vi "Read XML_Parse BC messageBuffers.vi"(8 "error in (no error)":errorcluster, 10 "channel in":T1, 11 "busController in":refnum<k24>) -> (0 "error out":errorcluster, 2 "channel out":T1, 3 "busController out":refnum<k24>)   [LabVIEW 2020, in "Ballard 1553 System Explorer.lvlib"]
uses:
  Ballard 1553 System Explorer.lvlib
  Ballard_Channel.ctl
  Ballard_BC.ctl
  Ballard_message.ctl
  Ballard_messageType.ctl
  Ballard_CWD1.ctl
  Ballard_CWD2.ctl
  Ballard_minorFrame.ctl
  Ballard_majorFrame.ctl
  Ballard_acyclicFrame.ctl
  Ballard_RT.ctl
  Ballard_RT subAddress.ctl
  Ballard_RT direction.ctl
  Ballard_RT rtMode.ctl
  Ballard_RT modeCode.ctl
  C:/Users/Administrator/Desktop/GIT/Ballard-MIL-STD-1553-Custom-Device/Source/System Explorer/SubVIs/Parse XML Ballard/1.2/BTIXML_SerDes.dll
  1.2/BTIXML_SerDes.dll
  Shared/Controls and Global/Global.vi
  Shared/Ballard 1553 Shared.lvlib
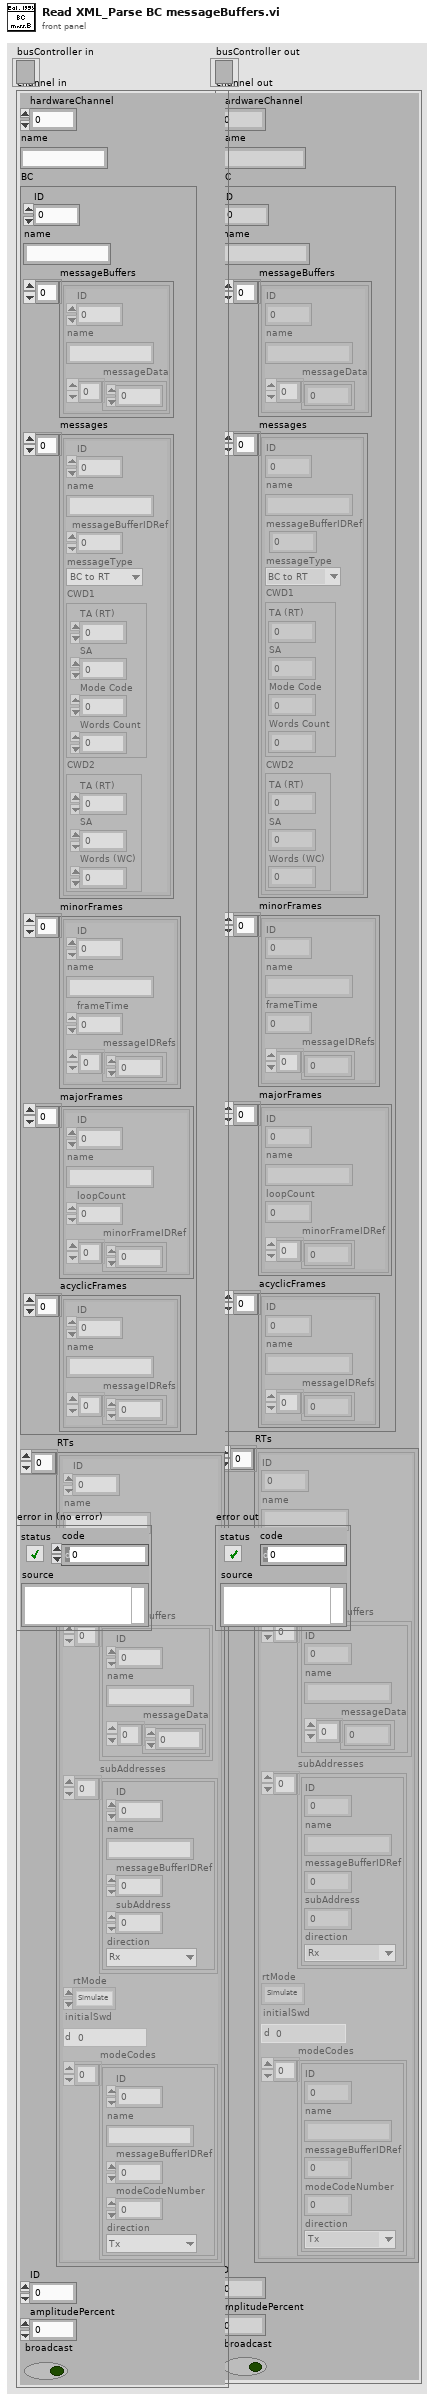
[diagram p1: front panel]
types:
  T1 = typedef "Ballard 1553 System Explorer.lvlib/Ballard_Channel.ctl" = cluster{"hardwareChannel":i32, "name":string, "BC":T2, "RTs":T10[], "ID":i32, "amplitudePercent":dbl, "broadcast":bool}
  T2 = typedef "Ballard 1553 System Explorer.lvlib/Ballard_BC.ctl" = cluster{"ID":i32, "name":string, "messageBuffers":cluster{"ID":i32, "name":string, "messageData":u16[]}[], "messages":T3[], "minorFrames":T7[], "majorFrames":T8[], "acyclicFrames":T9[]}
  T3 = typedef "Ballard 1553 System Explorer.lvlib/Ballard_message.ctl" = cluster{"ID":i32, "name":string, "messageBufferIDRef":i32, "messageType":T4, "CWD1":T5, "CWD2":T6}
  T4 = typedef "Ballard 1553 System Explorer.lvlib/Ballard_messageType.ctl" = enum16{"BC to RT", "RT to BC", "RT to RT", "MC (Rx)", "MC (Tx)"}
  T5 = typedef "Ballard 1553 System Explorer.lvlib/Ballard_CWD1.ctl" = cluster{"TA (RT)":i8, "SA":i8, "Mode Code":i8, "Words Count":i8}
  T6 = typedef "Ballard 1553 System Explorer.lvlib/Ballard_CWD2.ctl" = cluster{"TA (RT)":i8, "SA":i8, "Words (WC)":i8}
  T7 = typedef "Ballard 1553 System Explorer.lvlib/Ballard_minorFrame.ctl" = cluster{"ID":i32, "name":string, "frameTime":i32, "messageIDRefs":i32[]}
  T8 = typedef "Ballard 1553 System Explorer.lvlib/Ballard_majorFrame.ctl" = cluster{"ID":i32, "name":string, "loopCount":i32, "minorFrameIDRef":i32[]}
  T9 = typedef "Ballard 1553 System Explorer.lvlib/Ballard_acyclicFrame.ctl" = cluster{"ID":i32, "name":string, "messageIDRefs":i32[]}
  T10 = typedef "Ballard 1553 System Explorer.lvlib/Ballard_RT.ctl" = cluster{"ID":i32, "name":string, "rtAddress":i8, "responseTime":i32, "messageBuffers":cluster{"ID":i32, "name":string, "messageData":u16[]}[], "subAddresses":T11[], "rtMode":T13, "initialSwd":u16, "modeCodes":T14[]}
  T11 = typedef "Ballard 1553 System Explorer.lvlib/Ballard_RT subAddress.ctl" = cluster{"ID":i32, "name":string, "messageBufferIDRef":i32, "subAddress":i8, "direction":T12}
  T12 = typedef "Ballard 1553 System Explorer.lvlib/Ballard_RT direction.ctl" = enum16{"Tx", "Rx"}
  T13 = typedef "Ballard 1553 System Explorer.lvlib/Ballard_RT rtMode.ctl" = enum16{"Simulate", "Monitor", "Disable"}
  T14 = typedef "Ballard 1553 System Explorer.lvlib/Ballard_RT modeCode.ctl" = cluster{"ID":i32, "name":string, "messageBufferIDRef":i32, "modeCodeNumber":i8, "direction":T12}
  T15 = cluster{"ID":i32, "name":string, "messageData":u16[]}
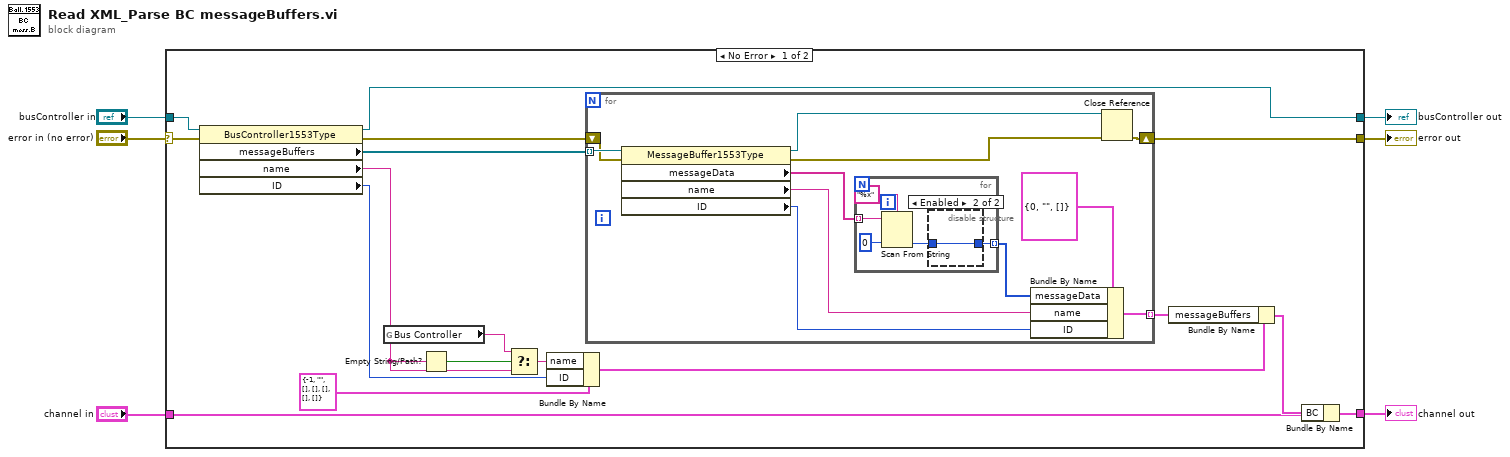
[diagram p0: block diagram]
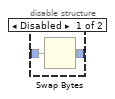
[diagram p2: hidden frame]
diagram:
  n1 = case shown="No Error" "error in (no error)" {
    selector: "error in (no error)" -> [w11 w45]
    tunnel: [w23 w43] -> w6
    tunnel: "channel in" -> [w21 w43]
    tunnel: [w20 w45] -> w4
    tunnel: [w19 w44] -> w3
    tunnel: "busController in" -> [w12 w44]
    frame No Error {
      n2 = property class="BusController1553Type"(reference=w12, error in=w11) -> (reference out=w19:refnum<k24>, error out=w14:errorcluster, "messageBuffers"=w13:refnum<k24>[], "name"=w9:string, "ID"=w16:i32)
      n3 = global read "Global.vi" "Bus Controller"() -> (w7:string)
      n4 = Empty String/Path?(string/path=w9) -> (empty?=w10:bool)
      n5 = Select(t=w7, s=w10, f=w9) -> (s? t:f=w8:string)
      n6 = Bundle By Name(cluster=T2 {"ID"=-1, "name"="", "messageBuffers"=[], "messages"=[], "minorFrames"=[], "majorFrames"=[], "acyclicFrames"=[]} ("BC"), "name"=w8, "ID"=w16) -> (w17:T2)
      n7 = for {
        tunnel: w13 -> [w34] mode=indexing
        shift-right: [w31] -> w20
        shift-left: w14 -> [w33]
        tunnel: [w24] -> w18 mode=indexing
        n8 = property class="MessageBuffer1553Type"(reference=w34, error in=w33) -> (reference out=w32:refnum<k24>, error out=w30:errorcluster, "messageData"=w29:string[], "name"=w26:string, "ID"=w25:i32)
        n9 = for {
          tunnel: w29 -> [w39] mode=indexing
          tunnel: [w35] -> w27 mode=indexing
          n10 = Scan From String(format string="%x", input string=w39, default 1=u16 0) -> (output 1=w36:u16)  [unwired: 2 in, 3 out]
          n11 = disable-structure shown="Enabled" {
            disable-tunnel: w36 -> [w41 w42]
            disable-tunnel: [w40 w42] -> w35
            frame Disabled {
              n12 = Swap Bytes(anything=w41) -> (byte swapped=w40:u16)
            }
            frame Enabled {
            }
          }
        }
        n13 = Bundle By Name(cluster=T15 {"ID"=0, "name"="", "messageData"=[]} ("messageBuffer"), "messageData"=w27, "name"=w26, "ID"=w25) -> (w24:T15)
        n14 = Close Reference(reference=w32, error in (no error)=w30) -> (error out=w31:errorcluster)
      }
      n15 = Bundle By Name(cluster=w17, "messageBuffers"=w18) -> (w22:T2)
      n16 = Bundle By Name(cluster=w21, "BC"=w22) -> (w23:T1)
    }
    frame Error {
    }
  }
  "channel out" <- w6
  "error out" <- w4
  "busController out" <- w3
